vi "FlushQueue.vi"(8 "error in":errorcluster) -> (0 "error out":errorcluster)   [LabVIEW 2018, in "S5.lvclass"]
uses:
  S5.lvclass
  Queue/Queue Data.ctl
  Queue/State.ctl
panel:
  out "remaining elements":T1[](array[typedef])
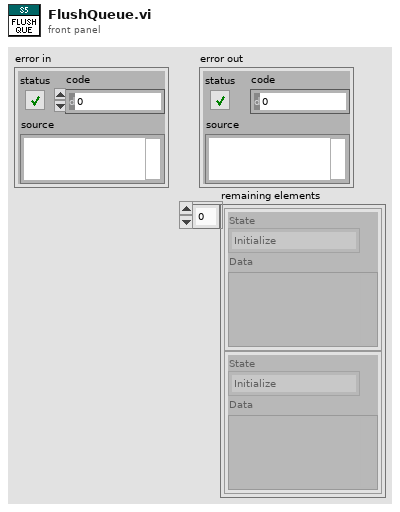
[diagram p1: front panel]
types:
  T1 = typedef "S5.lvclass/Queue Data.ctl" = cluster{"State":T2, "Data":variant}
  T2 = typedef "S5.lvclass/State.ctl" = enum16{"Initialize", "SetConfig", "AckAlarm", "Alarm", "Idle", "LockLid", "LowPressure", "Pressurize", "DecayTest", "Vent", "Abort", "Start", "CreateReports", "WriteToReport", "WritePressure", "Error", "Exit"}
  T3 = typedef "S2.lvclass/Queue Data.ctl" = cluster{"State":T4, "Data":variant}
  T4 = typedef "S2.lvclass/State.ctl" = enum16{"Initialize", "SetConfig", "AckAlarm", "Alarm", "Idle", "LockLid", "LowPressure", "Pressurize", "DecayTest", "Vent", "Abort", "Start", "CreateReports", "WriteToReport", "WritePressure", "Error", "Exit"}
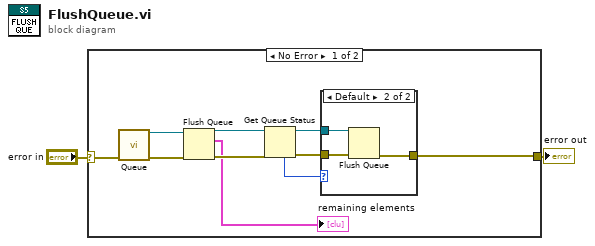
[diagram p0: block diagram]
diagram:
  n1 = case shown="No Error" "error in" {
    selector: "error in" -> [w12 w17]
    tunnel: [w5 w17] -> w2
    frame No Error {
      n2 = call "Queue.vi"("error in"=w12) -> ("error out"=w10:errorcluster, "queue out"=w11:refnum<queue>)  [unwired: 9 in]
      n3 = Flush Queue(queue=w11, error in (no error)=w10) -> (queue out=w8:refnum<queue>, remaining elements=→"remaining elements":T3[], error out=w9:errorcluster)
      n4 = Get Queue Status(queue=w8, error in (no error)=w9) -> (queue out=w7:refnum<queue>, error out=w6:errorcluster, # elements in queue=w4:i32)  [unwired: 1 in, 5 out]
      n5 = case shown="Default" w4 {
        tunnel: w7 -> [_ w16]
        tunnel: w6 -> [w13 w15]
        tunnel: [w13 w14] -> w5
        frame 0 {
        }
        frame Default {
          n6 = Flush Queue(queue=w16, error in (no error)=w15) -> (error out=w14:errorcluster)  [unwired: 2 out]
        }
      }
    }
    frame Error {
    }
  }
  "error out" <- w2
